vi "Read Icon Data from Library.vi"(10 "Default body text":T2 {"Body Text Spec"."Alignment" items=["left", "center", "right"]}, 11 "Library in":refnum<vi>) -> (2 "Data":T1={"Text Visible?"=FALSE, "Text Opacity"=0, "Templ Visible?"=FALSE, "Templ Opacity"=0, "Relative Path from 1 to 2"=path "", "Image"=bytes[0], "All User Layers"=[], "Body Text"={"Line 1 text"="", "Line 2 text"="", "Line 3 text"="", "Line 4 text"="", "Line 1 color"=0, "Line 2 color"=0, "Line 3 color"=0, "Line 4 color"=0, "Body Text Spec"={"Font"="", "Alignment"=0, "Size"=3}, "Center text vertically"=FALSE, "Capitalize Text"=FALSE}} {"Body Text"."Body Text Spec"."Alignment" items=["left", "center", "right"]}, 3 "Library out":refnum<vi>)   [LabVIEW 2020, in "lv_icon.lvlib"]
doc: "Read LabVIEW Icon Data from a Library."
uses:
  resource/plugins/lv_icon.lvlib
  Classes/Layer/Layer.lvclass
  Controls/Font.ctl
  Controls/Alignment.ctl
  Controls/BodyText.ctl
  Controls/LabVIEW Icon Stored Information.ctl
panel:
  out "error out":errorcluster
  in  "error in":errorcluster
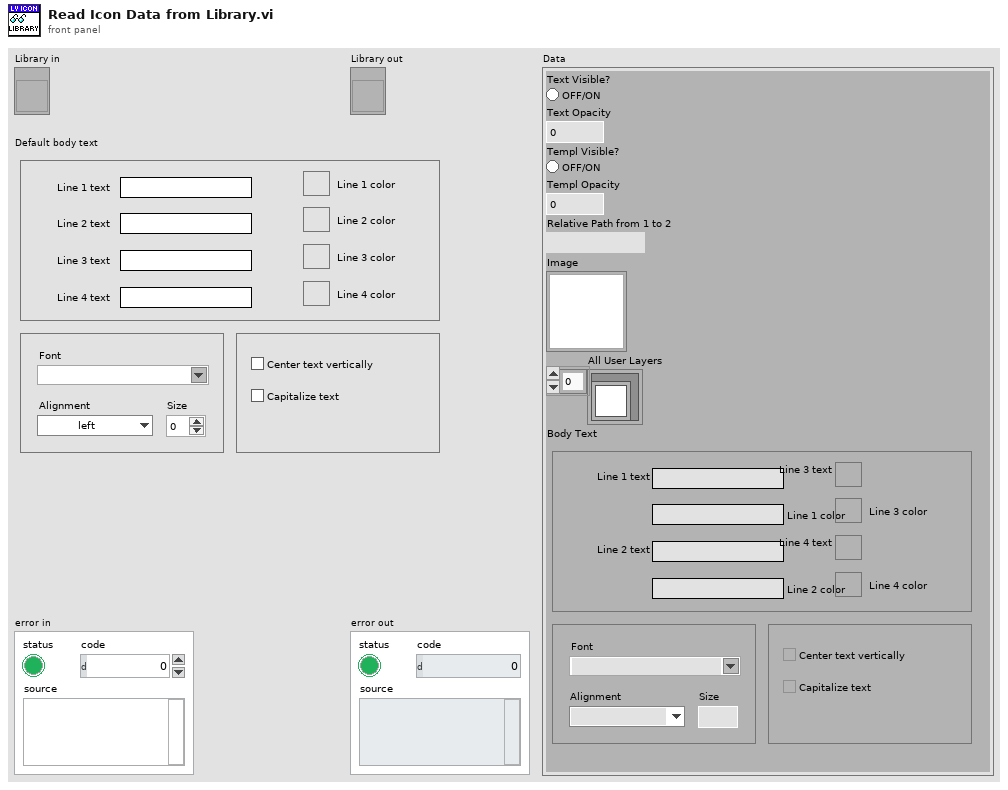
[diagram p1: front panel]
types:
  T1 = typedef "LabVIEW Icon Stored Information.ctl" = cluster{"Text Visible?":bool, "Text Opacity":u8, "Templ Visible?":bool, "Templ Opacity":u8, "Relative Path from 1 to 2":path, "Image":picture, "All User Layers":refnum<class "Layer.lvclass">[], "Body Text":T2}
  T2 = typedef "BodyText.ctl" = cluster{"Line 1 text":string, "Line 2 text":string, "Line 3 text":string, "Line 4 text":string, "Line 1 color":u32, "Line 2 color":u32, "Line 3 color":u32, "Line 4 color":u32, "Body Text Spec":cluster{"Font":T3, "Alignment":T4, "Size":u8}, "Center text vertically":bool, "Capitalize Text":bool}
  T3 = typedef "Font.ctl" = string
  T4 = typedef "Alignment.ctl" = u16
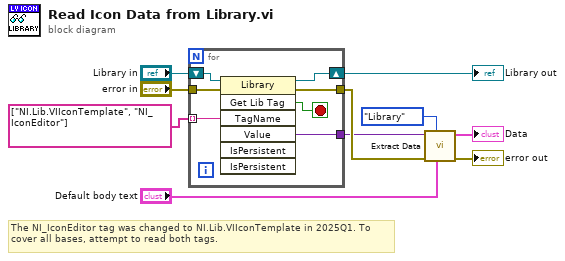
[diagram p0: block diagram]
diagram:
  # "The NI_IconEditor tag was changed to NI.Lib.VIIconTemplate in 2025Q1. To cover all bases, attempt to read both tags."
  n1 = for {
    tunnel: [w15] -> w5
    shift-right: [w14] -> w4
    shift-left: "Library in" -> [w13]
    tunnel: string[] ["NI.Lib.VIIconTemplate", "NI_IconEditor"] -> [w11] mode=indexing
    tunnel: "error in" -> [w16]
    tunnel: [w17] -> w10
    stop <- w12 stop-if-true
    n2 = invoke class="Library" method="Get Lib Tag"(reference=w13, error in=w16, "TagName"=w11) -> (reference out=w14:refnum<vi>, error out=w17:errorcluster, "GetTag"=w12:bool, "Value"=w15:variant)  [unwired: 4 in, 3 out]
  }
  "Library out" <- w4
  n3 = call "Extract Data.vi"("Default body text"="Default body text", "Type"=enum16{"VI", "Library"}."Library", "error in"=w10, "Value"=w5) -> ("error out"=→"error out":errorcluster, "Data"=→"Data":T1)  [unwired: 6 out]
